vi "Result_Test.vi"(8 "error in (no error)":errorcluster caption="entrée d'erreur (pas d'erreur)", 11 "Delay en entrée":refnum<class "Enter_Qr_P2056.lvclass">) -> (0 "error out":errorcluster caption="sortie d'erreur", 3 "Delay en sortie":refnum<class "Enter_Qr_P2056.lvclass">)   [LabVIEW 2020, in "Library Test.lvlib" / "Enter_Qr_P2056.lvclass"]
uses:
  Enter_Qr_P2056.lvclass
  C:/Users/ngarcin/OneDrive - Altyor/Standard TB/Class/Test/Test (Default)/Test (Default).lvclass
  Test_Without_Instr/Test_Without_Inst.lvclass
  Enter_Qr_P2056.lvclass/Enter_Qr_P2056.ctl
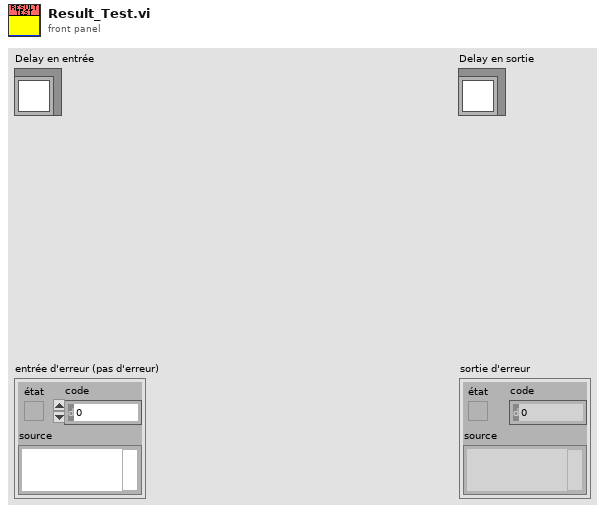
[diagram p1: front panel]
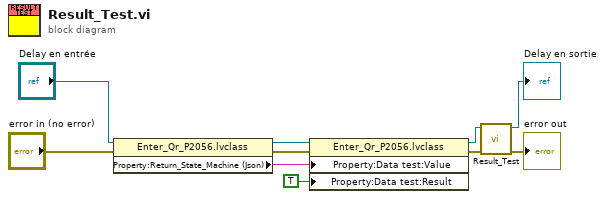
[diagram p0: block diagram]
diagram:
  n1 = property class="Enter_Qr_P2056.lvclass"(reference="Delay en entrée", error in="error in (no error)") -> (reference out=w5:refnum<class "Enter_Qr_P2056.lvclass">, error out=w3:errorcluster, "Property:Return_State_Machine (Json)"=w6:string)
  n2 = property class="Enter_Qr_P2056.lvclass"(reference=w5, error in=w3, "Property:Data test:Value"=w6, "Property:Data test:Result"=TRUE ("Result")) -> (reference out=w4:refnum<class "Enter_Qr_P2056.lvclass">, error out=w2:errorcluster)
  n3 = call-parent "Result_Test.vi"("error in (no error)"=w2, "Test_Without_Inst en entrée"=w4) -> ("error out"=→"error out":errorcluster, "Test_Without_Inst en sortie"=→"Delay en sortie":refnum<class "Enter_Qr_P2056.lvclass">)  [unwired: 8 in]
